vi "ETRONMTDaily.vi"() -> ()   [LabVIEW 2012]
uses:
  <vilib>/Utility/NIReport.llb/NI_report.lvclass
  <vilib>/addons/database/Connection.llb/DB Tools Open Connec (Path).vi
  <vilib>/addons/database/_DB Variant To Data/Database Variant To Data.xnode
  <vilib>/Utility/SMTP/NI_SMTPEmail.lvlib
  <vilib>/addons/database/NI_Database_API.lvlib
panel:
  out "error out 3":errorcluster
  out "appended path 2":path
  out "appended path":path
  out "data":string
  out "error out":errorcluster
  out "error out 2":errorcluster
  in  "MIME content-type (application/octet-stream)":string="application/octet-stream"
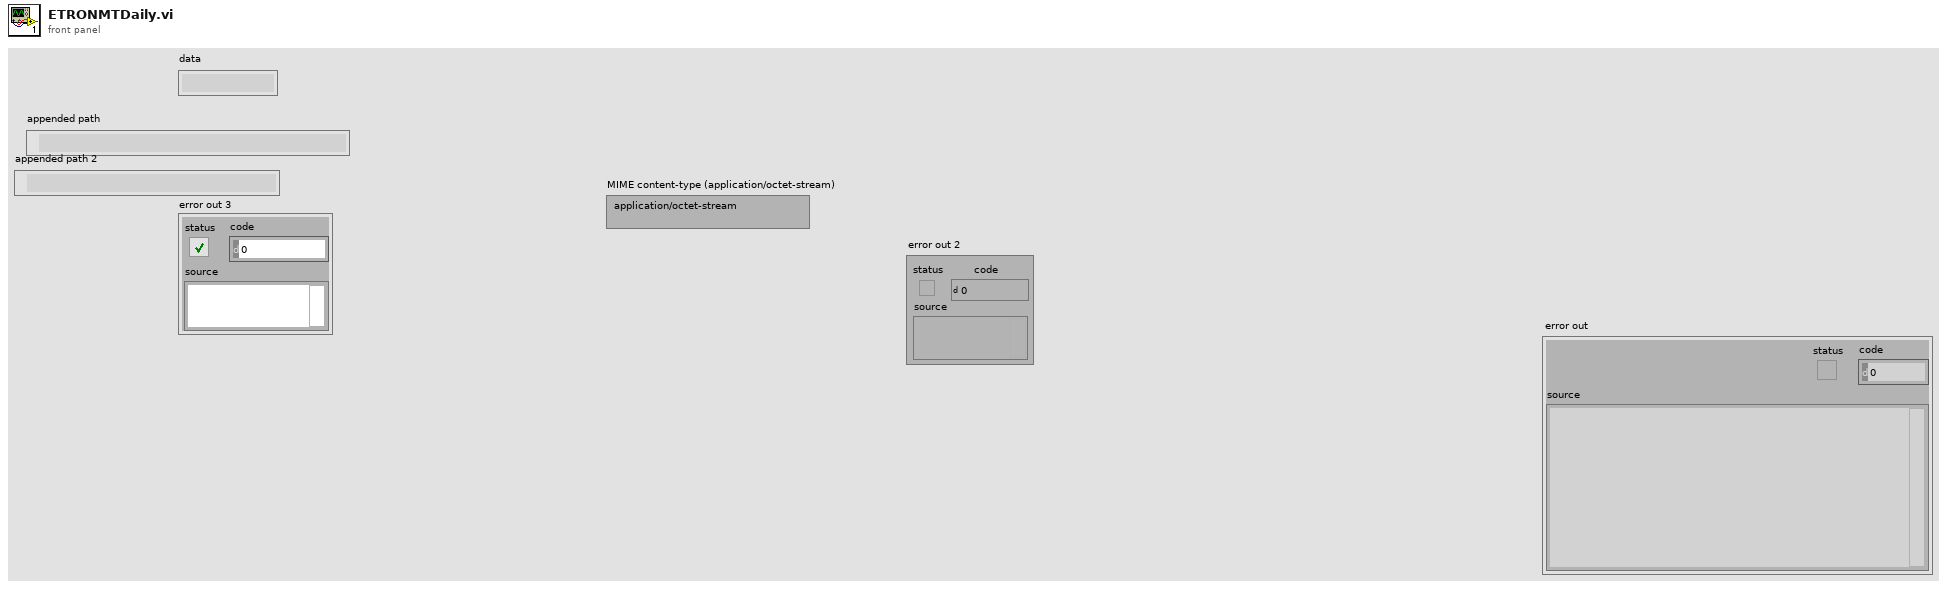
[diagram p1: front panel]
types:
  T1 = enum16{"Standard Report", "HTML", "Word", "Excel"}
  T2 = typedef "NI_Database_API.lvlib/Conn ObjectReference.ctl" = refnum<k1>
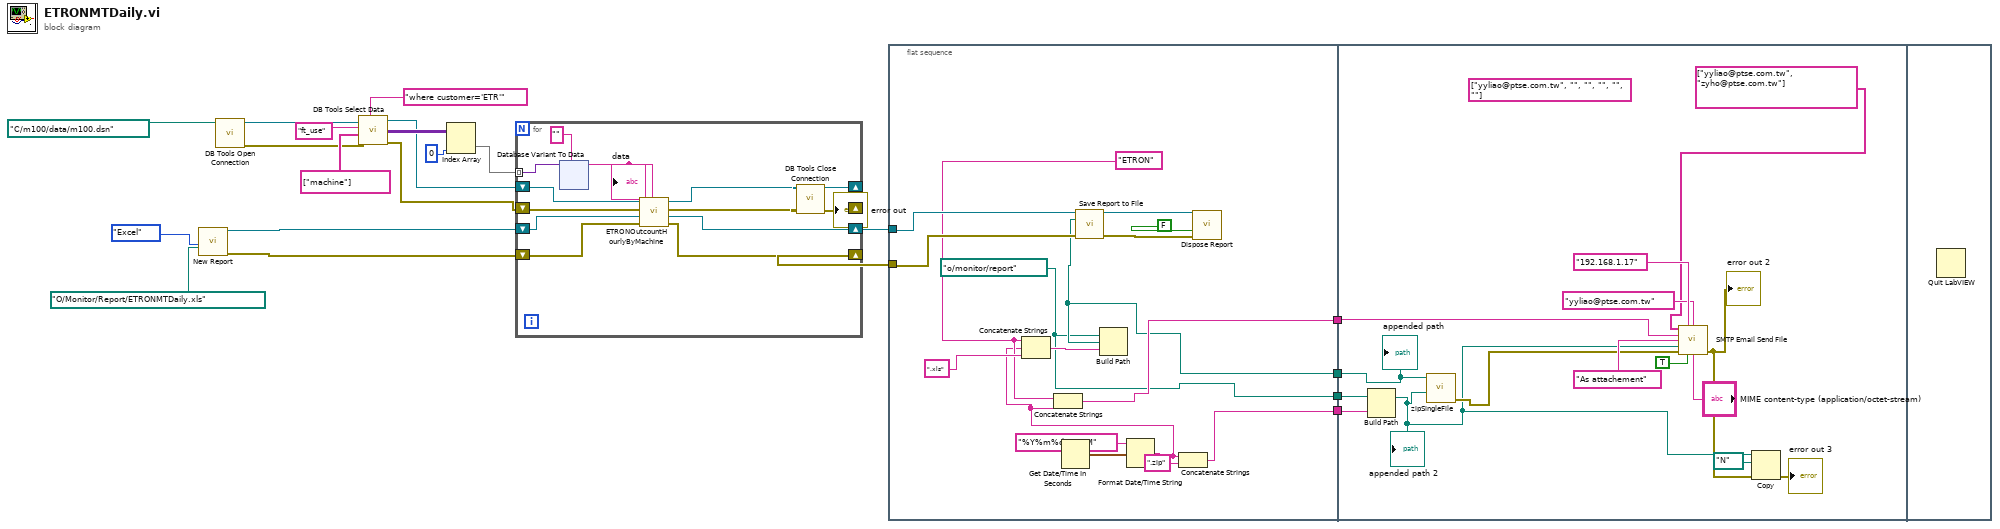
[diagram p0: block diagram]
diagram:
  n1 = call <vilib>:"New Report.vi"("report type"=T1."Excel" ("Report Type"), "template (empty)"=path "O:/Monitor/Report/ETRONMTDaily.xls") -> ("report out"=w5:refnum<class "NI_report.lvclass">, "error out"=w4:errorcluster)  [unwired: 12 in]
  n2 = call-poly <vilib>:"DB Tools Open Connection.vi"("connection information"=path "C:/m100/data/m100.dsn") -> ("error out"=w6:errorcluster, "connection reference"=w7:T2)  [unwired: 7 in]
  n3 = call <vilib>:"DB Tools Select Data.vi"("condition"="where customer='ETR'", "error in (no error)"=w6, "columns"=string[] ["machine"], "table"="ft_use", "connection reference"=w7) -> ("error out"=w14:errorcluster, "data"=w18:variant[][], "connection reference out"=w15:T2)  [unwired: 1 in]
  n4 = Index Array(array=w18, index (col)=0 ("disabled index (col)")) -> (element=w17:variant[])  [unwired: 1 in]
  n5 = for {
    tunnel: w17 -> [w34] mode=indexing
    shift-right: [w28] -> w12
    shift-left: w15 -> [w26]
    shift-right: [w27] -> w11
    shift-left: w14 -> [w25]
    shift-right: [w31] -> w10
    shift-left: w5 -> [w35]
    shift-right: [w30] -> w9
    shift-left: w4 -> [w29]
    n6 = xnode "Database Variant To Data"("database variant"=w34, "type"="") -> ("data"=w32:string)  [unwired: 1 in, 1 out]
    "data" <- w32
    n7 = call "ETRONOutcountHourlyByMachine.vi"("Machine"=w32, "error in (no error) 2"=w29, "report in"=w35, "error in (no error)"=w25, "connection reference"=w26) -> ("error in (no error) 3"=w30:errorcluster, "report in 2"=w31:refnum<class "NI_report.lvclass">, "error out"=w27:errorcluster, "connection reference 2"=w28:T2)  [unwired: 3 in]
  }
  n8 = call <vilib>:"DB Tools Close Connection.vi"("error in (no error)"=w11, "connection reference"=w12) -> ("error out"=→"error out":errorcluster)  [unwired: 5 in]
  n9 = flat-sequence {
    tunnel: w10 -> [w80]
    tunnel: w9 -> [w79]
    tunnel: [w75] -> w24
    tunnel: [w70] -> w3
    tunnel: [w69] -> w2
    tunnel: [w68] -> w1
    tunnel: w24 -> [w93]
    tunnel: w3 -> [w90]
    tunnel: w2 -> [w92]
    tunnel: w1 -> [w91]
    frame #0 {
      w76 = "ETRON" ("string")
      w69 = path "o:/monitor/report" ("base path")
      n10 = Get Date/Time In Seconds() -> (seconds since 1Jan1904=w74:timestamp)
      n11 = Format Date/Time String(time format string (%c)="%Y%m%d%H%M", seconds (now)=w74) -> (date/time string=w71:string)  [unwired: 1 in]
      n12 = Concatenate Strings(w76, w71, ".xls" ("string")) -> (w77:string)
      n13 = Concatenate Strings(w76, w71) -> (w75:string)
      n14 = Build Path(base path=w69, name or relative path=w77) -> (appended path=w70:path)
      n15 = call-dynamic "Save Report to File.vi"("report in"=w80, "report file path"=w70, "error in (no error)"=w79) -> ("report out"=w82:refnum<class "NI_report.lvclass">, "error out"=w81:errorcluster)  [unwired: 11 in]
      n16 = Concatenate Strings(w71, ".zip" ("string")) -> (w68:string)
      n17 = call-dynamic "Dispose Report.vi"("report in"=w82, "save changes? (F)"=FALSE, "error in (no error)"=w81) -> ()  [unwired: 12 in, 1 out]
    }
    frame #1 {
      (unwired) string[] ["yyliao@ptse.com.tw", "", "", "", "", ""] ("recipients")
      n18 = Build Path(base path=w92, name or relative path=w91) -> (appended path=w88:path)
      "appended path 2" <- w88
      n19 = call "zipSingleFile.vi"("zip folderFile"=w88, "source file path"=w90) -> ("error out"=w89:errorcluster)  [unwired: 9 in]
      n20 = call <vilib>:"SMTP Email Send File.vi"("recipients"=string[] ["yyliao@ptse.com.tw", "zyho@ptse.com.tw"], "mail server"="192.168.1.17", "return address"="yyliao@ptse.com.tw", "subject ([No Subject])"=w93, "message"="As attachement", "file path"=w88, "error in (no error)"=w89, "binary? (F)"=TRUE, "MIME content-type (application/octet-stream)"="MIME content-type (application/octet-stream)") -> ("error out"=w85:errorcluster)  [unwired: 5 in, 1 out]
      "error out 2" <- w85
      n21 = Copy(8:w85, 10:path "N:/" ("target path (use dialog)"), 11:w88) -> (0:→"error out 3":errorcluster)  [unwired: 2 in, 2 out]
      "appended path" <- w90
    }
    frame #2 {
      n22 = Quit LabVIEW() -> ()  [unwired: 1 in]
    }
  }
